vi "Save Image Crop.vi"(8 "error in (no error)":errorcluster, 11 "Frame Grabber Data In":T1={"Camera Session"="", "Frame"=refnum, "AVI Refnum"=refnum, "Codecs"=[], "Frame number"=0, "Tracking File Refnum"=refnum, "Tick Count"=0, "Probe Object"=refnum, "Playback Probe Data"=[], "Rigid Body"={"Position"={"x (mm)"=0.0, "y (mm)"=0.0, "z (mm)"=0.0}, "Orientation"={"Pitch (rad)"=0.0, "Yaw (rad)"=0.0, "Roll (rad)"=0.0}, "Quaternion"={"qx"=0.0, "qy"=0.0, "qz"=0.0, "qw"=0.0}, "Tracked?"=FALSE}, "Total no frames playback"=0, "Video FPS"=0.0, "Camera connected?"=FALSE, "Scene"=refnum, "Cropped Frame"=refnum, "Tracker FPS"=0.0, "Crop ROI"=[], "Presentation Values"=[], "Elapsed time (ms)"=0, "Camera frames playback"=0, "Refnums"={"Live Refnum"=refnum, "Record Refnum"=refnum, "Playback Refnum"=refnum, "Frame Slider Refnum"=refnum, "Pause Refnum"=refnum, "Home Refnum"=refnum, "Set Crop Refnum"=refnum, "Clear Crop Refnum"=refnum, "stop refnum"=refnum, "Playback Rate Refnum"=refnum, "Presentation Refnum"=refnum, "Crop Time Frame Slider Refnum"=refnum, "Cancel Save Refnum"=refnum, "Reverse Playback Refnum"=refnum, "Recording Settings Refnum"=refnum, "Continuous Playback Refnum"=refnum, "Annotation Refnum"=refnum, "Export All Refnum"=refnum, "Export List Refnum"=refnum, "Fill List Refnum"=refnum, "Save Crop Refnum"=refnum, "Skip Forward Refnum"=refnum, "Skip Backward Refnum"=refnum, "Single Annotation Refnum"=refnum, "Load Video Refnum"=refnum, "Set Start Refnum"=refnum, "Set End Refnum"=refnum, "Add to List Refnum"=refnum, "List of Annotations Refnum"=refnum, "Camera Frame Refnum"=refnum, "Load Image Refnum"=refnum, "Saving Refnum"=refnum}, "Dimensions"={"Probe Dimensions"={"Probe Width"=0.0, "Probe Depth"=1.0, "Probe Height"=0.0}, "Room Dimensions"={"Room Width"=0.0, "Room Depth"=0.0, "Room Height"=0.0}}, "Playback Data As Strings"=[], "Cropped Tracking File Refnum"=refnum, "Cropped AVI Refnum"=refnum, "Header"=[], "Total euclidian distance"=0.0, "Annotation File Path"=path "", "Playback File Path"=path "", "Size per frame"=0.0, "Ground Truth File Refnum"=refnum, "Annotation Array"=[], "Annotation TIFFs Folder"=path "", "overwriting open file?"=FALSE, "Image Sequence"=[], "Video/Image Flag"=enum."Playback Video Frame", "Image sequence?"=FALSE, "Image sequence filenames"=[]}) -> (0 "error out":errorcluster, 3 "Frame Grabber Data Out":T1={"Camera Session"="", "Frame"=refnum, "AVI Refnum"=refnum, "Codecs"=[], "Frame number"=0, "Tracking File Refnum"=refnum, "Tick Count"=0, "Probe Object"=refnum, "Playback Probe Data"=[], "Rigid Body"={"Position"={"x (mm)"=0.0, "y (mm)"=0.0, "z (mm)"=0.0}, "Orientation"={"Pitch (rad)"=0.0, "Yaw (rad)"=0.0, "Roll (rad)"=0.0}, "Quaternion"={"qx"=0.0, "qy"=0.0, "qz"=0.0, "qw"=0.0}, "Tracked?"=FALSE}, "Total no frames playback"=0, "Video FPS"=0.0, "Camera connected?"=FALSE, "Scene"=refnum, "Cropped Frame"=refnum, "Tracker FPS"=0.0, "Crop ROI"=[], "Presentation Values"=[], "Elapsed time (ms)"=0, "Camera frames playback"=0, "Refnums"={"Live Refnum"=refnum, "Record Refnum"=refnum, "Playback Refnum"=refnum, "Frame Slider Refnum"=refnum, "Pause Refnum"=refnum, "Home Refnum"=refnum, "Set Crop Refnum"=refnum, "Clear Crop Refnum"=refnum, "stop refnum"=refnum, "Playback Rate Refnum"=refnum, "Presentation Refnum"=refnum, "Crop Time Frame Slider Refnum"=refnum, "Cancel Save Refnum"=refnum, "Reverse Playback Refnum"=refnum, "Recording Settings Refnum"=refnum, "Continuous Playback Refnum"=refnum, "Annotation Refnum"=refnum, "Export All Refnum"=refnum, "Export List Refnum"=refnum, "Fill List Refnum"=refnum, "Save Crop Refnum"=refnum, "Skip Forward Refnum"=refnum, "Skip Backward Refnum"=refnum, "Single Annotation Refnum"=refnum, "Load Video Refnum"=refnum, "Set Start Refnum"=refnum, "Set End Refnum"=refnum, "Add to List Refnum"=refnum, "List of Annotations Refnum"=refnum, "Camera Frame Refnum"=refnum, "Load Image Refnum"=refnum, "Saving Refnum"=refnum}, "Dimensions"={"Probe Dimensions"={"Probe Width"=0.0, "Probe Depth"=1.0, "Probe Height"=0.0}, "Room Dimensions"={"Room Width"=0.0, "Room Depth"=0.0, "Room Height"=0.0}}, "Playback Data As Strings"=[], "Cropped Tracking File Refnum"=refnum, "Cropped AVI Refnum"=refnum, "Header"=[], "Total euclidian distance"=0.0, "Annotation File Path"=path "", "Playback File Path"=path "", "Size per frame"=0.0, "Ground Truth File Refnum"=refnum, "Annotation Array"=[], "Annotation TIFFs Folder"=path "", "overwriting open file?"=FALSE, "Image Sequence"=[], "Video/Image Flag"=enum."Playback Video Frame", "Image sequence?"=FALSE, "Image sequence filenames"=[]})   [LabVIEW 2017]
uses:
  Controls/Frame Grabber Data.ctl
  <vilib>/userdefined/High Color/IMAQdx.ctl
  <vilib>/vision/Image Controls.llb/IMAQ Image.ctl
  <vilib>/vision/Avi.llb/IMAQ AVI2 Refnum.ctl
  Controls/Rigid Body Info.ctl
  Controls/Position.ctl
  Controls/Orientation.ctl
  Controls/Refnums.ctl
  Controls/Recording Settings.ctl
  Controls/Operator Settings.ctl
  Controls/Operator.ctl
  Controls/Patient Settings.ctl
  Controls/Dimensions.ctl
  Controls/Room Dimensions.ctl
  Controls/Crop Video State.ctl
  <vilib>/vision/NI_Vision_Development_Module.lvlib
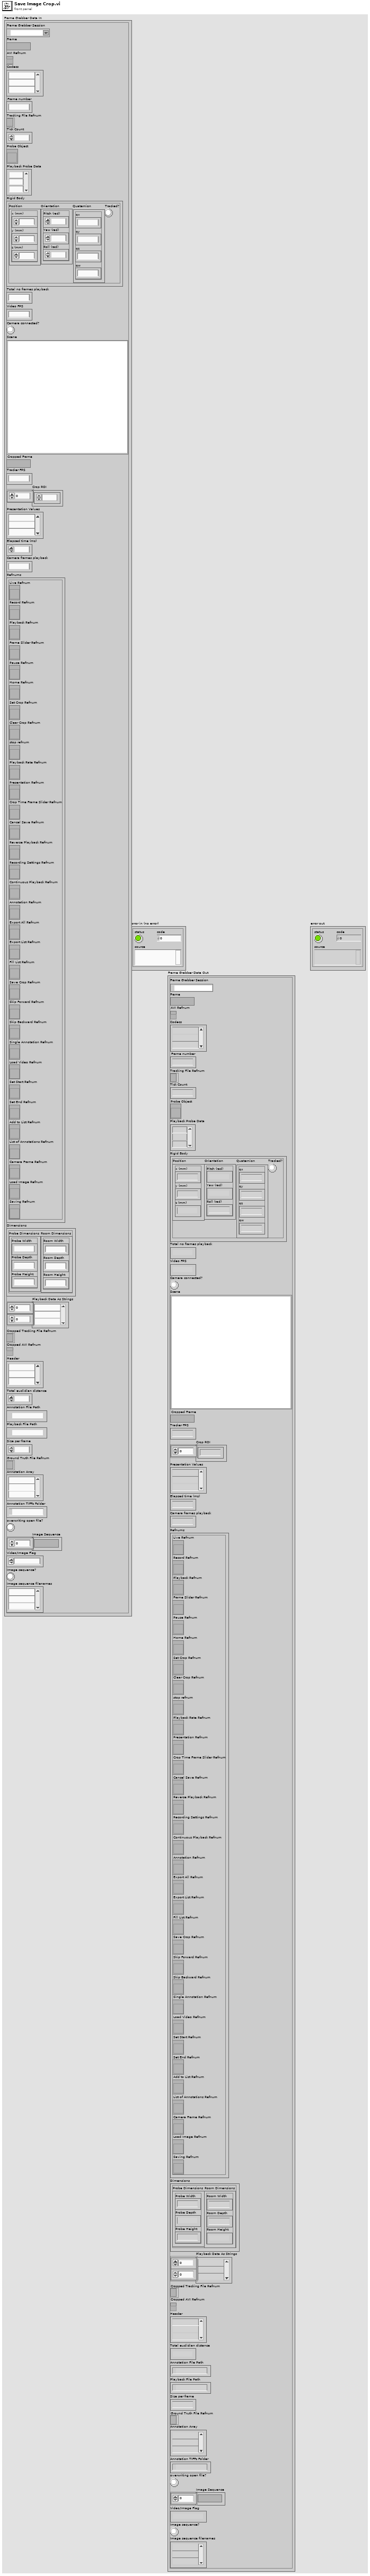
[diagram p1: front panel]
types:
  T1 = typedef "Frame Grabber Data.ctl" = cluster{"Camera Session":T2, "Frame":T3, "AVI Refnum":T4, "Codecs":string[], "Frame number":u32, "Tracking File Refnum":refnum<file>, "Tick Count":u32, "Probe Object":refnum<vi>, "Playback Probe Data":dbl[][], "Rigid Body":T5, "Total no frames playback":i32, "Video FPS":dbl, "Camera connected?":bool, "Scene":refnum<vi>, "Cropped Frame":T3, "Tracker FPS":dbl, "Crop ROI":i32[], "Presentation Values":string[], "Elapsed time (ms)":u32, "Camera frames playback":u32, "Refnums":T8, "Dimensions":T9, "Playback Data As Strings":string[][], "Cropped Tracking File Refnum":refnum<file>, "Cropped AVI Refnum":T4, "Header":string[], "Total euclidian distance":dbl, "Annotation File Path":path, "Playback File Path":path, "Size per frame":dbl, "Ground Truth File Refnum":refnum<file>, "Annotation Array":string[], "Annotation TIFFs Folder":path, "overwriting open file?":bool, "Image Sequence":T3[], "Video/Image Flag":T11, "Image sequence?":bool, "Image sequence filenames":string[]}
  T2 = typedef "IMAQdx.ctl" = refnum<k21>
  T3 = typedef "IMAQ Image.ctl" = refnum<image>
  T4 = typedef "IMAQ AVI2 Refnum.ctl" = refnum<k20>
  T5 = typedef "Rigid Body Info.ctl" = cluster{"Position":T6, "Orientation":T7, "Quaternion":cluster{"qx":sgl, "qy":sgl, "qz":sgl, "qw":sgl}, "Tracked?":bool}
  T6 = typedef "Position.ctl" = cluster{"x (mm)":sgl, "y (mm)":sgl, "z (mm)":sgl}
  T7 = typedef "Orientation.ctl" = cluster{"Pitch (rad)":sgl, "Yaw (rad)":sgl, "Roll (rad)":sgl}
  T8 = typedef "Refnums.ctl" = cluster{"Live Refnum":refnum<vi>, "Record Refnum":refnum<vi>, "Playback Refnum":refnum<vi>, "Frame Slider Refnum":refnum<vi>, "Pause Refnum":refnum<vi>, "Home Refnum":refnum<vi>, "Set Crop Refnum":refnum<vi>, "Clear Crop Refnum":refnum<vi>, "stop refnum":refnum<vi>, "Playback Rate Refnum":refnum<vi>, "Presentation Refnum":refnum<vi>, "Crop Time Frame Slider Refnum":refnum<vi>, "Cancel Save Refnum":refnum<vi>, "Reverse Playback Refnum":refnum<vi>, "Recording Settings Refnum":refnum<vi>, "Continuous Playback Refnum":refnum<vi>, "Annotation Refnum":refnum<vi>, "Export All Refnum":refnum<vi>, "Export List Refnum":refnum<vi>, "Fill List Refnum":refnum<vi>, "Save Crop Refnum":refnum<vi>, "Skip Forward Refnum":refnum<vi>, "Skip Backward Refnum":refnum<vi>, "Single Annotation Refnum":refnum<vi>, "Load Video Refnum":refnum<vi>, "Set Start Refnum":refnum<vi>, "Set End Refnum":refnum<vi>, "Add to List Refnum":refnum<vi>, "List of Annotations Refnum":refnum<vi>, "Camera Frame Refnum":refnum<vi>, "Load Image Refnum":refnum<vi>, "Saving Refnum":refnum<vi>}
  T9 = typedef "Dimensions.ctl" = cluster{"Probe Dimensions":cluster{"Probe Width":sgl, "Probe Depth":sgl, "Probe Height":sgl}, "Room Dimensions":T10}
  T10 = typedef "Room Dimensions.ctl" = cluster{"Room Width":dbl, "Room Depth":dbl, "Room Height":dbl}
  T11 = typedef "Crop Video State.ctl" = enum16{"Init", "Wait", "Load Image", "Load Video", "Play/Pause", "Playback Video Frame", "Display Image", "Save Image Sequence", "Save Video", "Export List", "Export All", "Close", "Set Crop Area", "Reset Crop Area", "Crop Inside", "Crop Outside", "Multi-Crop", "Re-Open Files", "Annotate Frame", "Annotate Clip", "Add to List", "Fill List", "Set Start", "Set End", "Error Handling", "Shutdown"}
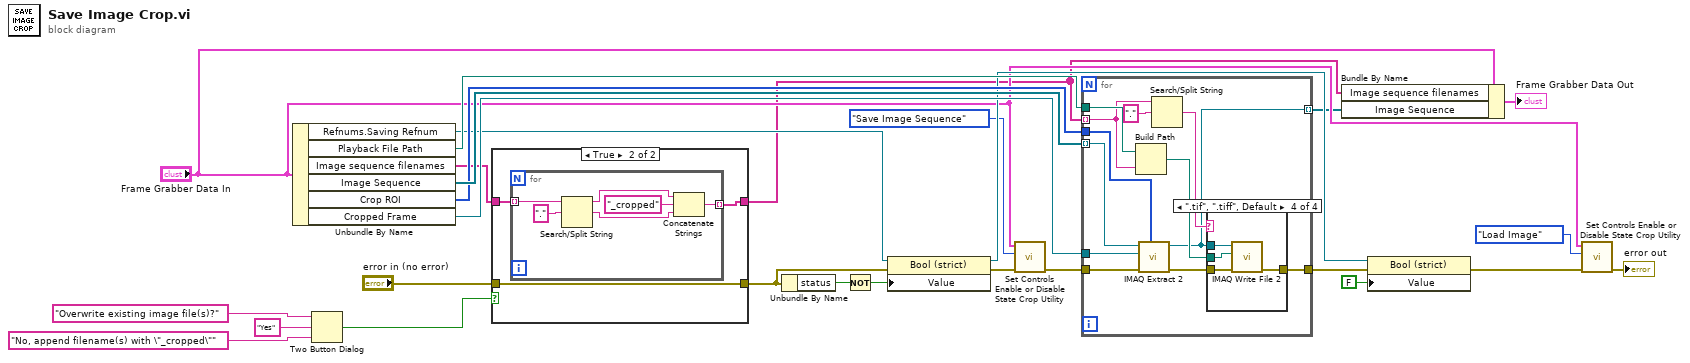
[diagram p0: block diagram]
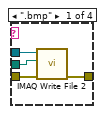
[diagram p3: hidden frame]
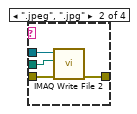
[diagram p4: hidden frame]
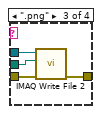
[diagram p5: hidden frame]
diagram:
  n1 = Unbundle By Name("Frame Grabber Data In") -> ("Refnums.Saving Refnum"=w17:refnum<vi>, "Playback File Path"=w24:path, "Image sequence filenames"=w18:string[], "Image Sequence"=w23:T3[], "Crop ROI"=w22:i32[], "Cropped Frame"=w21:T3)
  n2 = Two Button Dialog(message="Overwrite existing image file(s)?", 1:"No, append filename(s) with \"_cropped\"" ("F button name (\"Cancel\")"), 2:"Yes" ("T button name (\"OK\")")) -> (T button?=w20:bool)
  n3 = case shown="True" w20 {
    tunnel: [w29 w30] -> w16
    tunnel: "error in (no error)" -> [w29 w30]
    tunnel: [w28 w31] -> w2
    tunnel: w18 -> [w28 w32]
    frame False {
    }
    frame True {
      n4 = for {
        tunnel: w32 -> [w33] mode=indexing
        tunnel: [w34] -> w31 mode=indexing
        n5 = Search/Split String(string=w33, search string/char (-)=".") -> (substring before match=w38:string, match + rest of string=w37:string)  [unwired: 1 in, 1 out]
        n6 = Concatenate Strings(w38, "_cropped" ("string"), w37) -> (w34:string)
      }
    }
  }
  n7 = Unbundle By Name(w16) -> ("status"=w15:bool)
  n8 = Not(x=w15) -> (.not. x?=w14:bool)
  n9 = property class="Bool (strict)"(reference=w17, error in=w16, "Value"=w14) -> (reference out=w13:refnum<vi>, error out=w10:errorcluster)
  n10 = call "Set Controls Enable or Disable State Crop Utility.vi"("error in (no error)"=w10, "State"=Crop_Video_State."Save Image Sequence", "Frame Grabber Data In"="Frame Grabber Data In") -> ("error out"=w9:errorcluster)  [unwired: 8 in]
  n11 = for {
    tunnel: [w50] -> w12
    tunnel: w24 -> [w49]
    tunnel: w23 -> [w48] mode=indexing
    tunnel: w22 -> [w47]
    tunnel: w21 -> [w46]
    tunnel: w2 -> [w41] mode=indexing
    tunnel: w9 -> [w40]
    tunnel: [w39] -> w1 mode=indexing
    n12 = Build Path(base path=w49, name or relative path=w41) -> (appended path=w43:path)
    n13 = call "IMAQ Extract 2"("Optional Rectangle"=w47, "error in (no error)"=w40, "Image Dst"=w46, "Image Src"=w48) -> ("error out"=w42:errorcluster, "Image Dst Out"=w39:T3)  [unwired: 6 in]
    n14 = Search/Split String(string=w41, search string/char (-)=".") -> (match + rest of string=w45:string)  [unwired: 1 in, 2 out]
    n15 = case shown="\".tif\", \".tiff\", Default" w45 {
      tunnel: [w54 w58 w62 w66] -> w50
      tunnel: w43 -> [w53 w57 w61 w65]
      tunnel: w39 -> [w52 w56 w60 w63]
      tunnel: w42 -> [w51 w55 w59 w64]
      frame ".bmp" {
        n16 = call-poly "IMAQ Write File 2"("error in (no error)"=w51, "File Path"=w53, "Image"=w52) -> ("error out"=w54:errorcluster)  [unwired: 7 in, 1 out]
      }
      frame ".jpeg", ".jpg" {
        n17 = call-poly "IMAQ Write File 2"("error in (no error)"=w55, "File Path"=w57, "Image"=w56) -> ("error out"=w58:errorcluster)  [unwired: 7 in, 1 out]
      }
      frame ".png" {
        n18 = call-poly "IMAQ Write File 2"("error in (no error)"=w59, "File Path"=w61, "Image"=w60) -> ("error out"=w62:errorcluster)  [unwired: 7 in, 1 out]
      }
      frame ".tif", ".tiff", Default {
        n19 = call-poly "IMAQ Write File 2"("error in (no error)"=w64, "File Path"=w65, "Image"=w63) -> ("error out"=w66:errorcluster)  [unwired: 7 in, 1 out]
      }
    }
  }
  n20 = Bundle By Name(cluster="Frame Grabber Data In", "Image sequence filenames"=w2, "Image Sequence"=w1) -> (→"Frame Grabber Data Out":T1)
  n21 = property class="Bool (strict)"(reference=w13, error in=w12, "Value"=FALSE) -> (error out=w8:errorcluster)  [unwired: 1 out]
  n22 = call "Set Controls Enable or Disable State Crop Utility.vi"("error in (no error)"=w8, "State"=Crop_Video_State."Load Image", "Frame Grabber Data In"="Frame Grabber Data In") -> ("error out"=→"error out":errorcluster)  [unwired: 8 in]
